vi "Querry.vi"(8 "error in (no error)":errorcluster, 10 "PDU_req":T1={"Function Code"=1, "Data"=[], "RTU_DataBytes"=0}, 11 "MB_Master in":refnum<class "MB_Master.lvclass">) -> (0 "error out":errorcluster, 2 "PDU_resp":T1={"Function Code"=1, "Data"=[], "RTU_DataBytes"=0}, 3 "MB_Master out":refnum<class "MB_Master.lvclass">)   [LabVIEW 2016, in "MB Master.lvlib" / "MB_Master.lvclass"]
uses:
  MB_Master.lvclass
  MB_PDU/MB_PDU_Cluster.ctl
  MB Master.lvlib
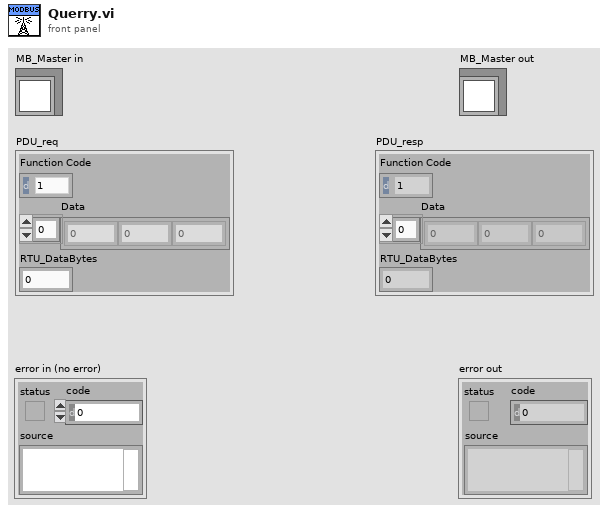
[diagram p1: front panel]
types:
  T1 = typedef "MB Master.lvlib/MB_PDU_Cluster.ctl" = cluster{"Function Code":u8, "Data":u8[], "RTU_DataBytes":i32}
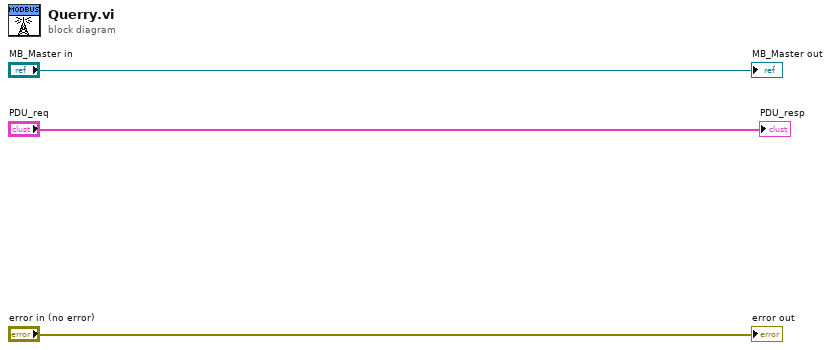
[diagram p0: block diagram]
diagram:
  "error out" <- "error in (no error)"
  "MB_Master out" <- "MB_Master in"
  "PDU_resp" <- "PDU_req"
